vi "ConvertTimes - Single.vi"(1 "GP22 Output":dbl) -> (0 "Time/s":dbl)   [LabVIEW 2018, in "GP22_TDC_Arduinoed.lvlib"]
doc: "Convert fixed point output of GP22 to time value in seconds. \n\nDepending on whether the TDC is in calibration mode or not, adjust the raw data by either the Ref clock's period (calibrated mode) or the calibration LSB time (uncalibrated mode)."
uses:
  GP22_TDC_Arduinoed.lvlib
  Public/Globals.vi
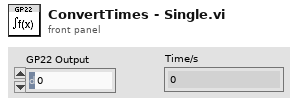
[diagram p1: front panel]
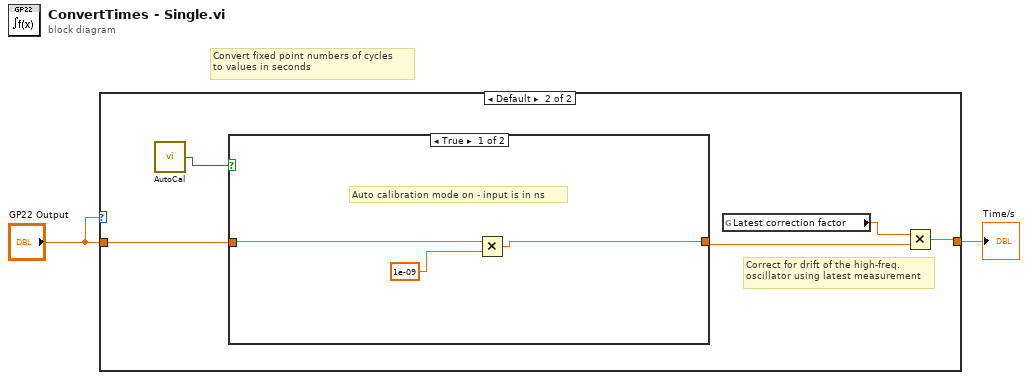
[diagram p0: block diagram]
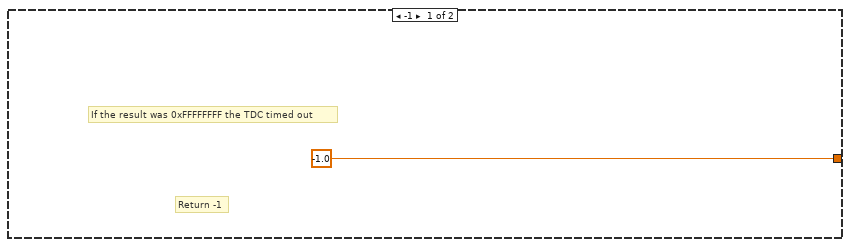
[diagram p2: hidden frame]
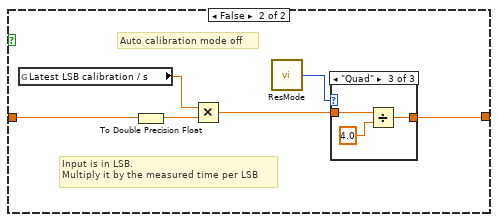
[diagram p3: hidden frame]
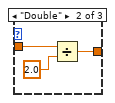
[diagram p5: hidden frame]
diagram:
  # "Convert fixed point numbers of cycles\nto values in seconds"
  n1 = case shown="Default" "GP22 Output" {
    tunnel: [-1.0 w5] -> w2
    tunnel: "GP22 Output" -> [_ w8]
    frame -1 {
      # "Return -1"
      # "If the result was 0xFFFFFFFF the TDC timed out"
    }
    frame Default {
      # "Correct for drift of the high-freq.\noscillator using latest measurement"
      n2 = call "AutoCal.vi"() -> ("Autocal mode?"=w7:bool)  [unwired: 2 in]
      n3 = case shown="True" w7 {
        tunnel: [w9 w14] -> w6
        tunnel: w8 -> [w10 w17]
        frame True {
          # "Auto calibration mode on - input is in ns"
          n4 = Multiply(x=w10, y=1e-09) -> (x*y=w9:dbl)
        }
        frame False {
          # "Input is in LSB. \nMultiply it by the measured time per LSB"
          # "Auto calibration mode off"
          n5 = global read "Globals.vi" "Latest LSB calibration / s"() -> (w15:dbl)
          n6 = To Double Precision Float(number=w17) -> (double precision float=w16:dbl)
          n7 = Multiply(x=w15, y=w16) -> (x*y=w13:dbl)
          n8 = call "ResMode.vi"() -> ("Resolution mode"=w12:enum16{"Single", "Double", "Quad"})  [unwired: 2 in]
          n9 = case shown="\"Quad\"" w12 {
            tunnel: [w18 w21 w24] -> w14
            tunnel: w13 -> [w18 w20 w23]
            frame "Single" {
            }
            frame "Double" {
              n10 = Divide(x=w20, y=2.0) -> (x/y=w21:dbl)
            }
            frame "Quad" {
              n11 = Divide(x=w23, y=4.0) -> (x/y=w24:dbl)
            }
          }
        }
      }
      n12 = global read "Globals.vi" "Latest correction factor"() -> (w4:dbl)
      n13 = Multiply(x=w4, y=w6) -> (x*y=w5:dbl)
    }
  }
  "Time/s" <- w2
